vi "intiStage.vi"() -> (0 "error out":errorcluster, 3 "VISA resource name out":refnum<visa-resource-name>)   [LabVIEW 2016]
uses:
  <vilib>/Instr/_visa.llb/VISA Configure Serial Port (Instr).vi
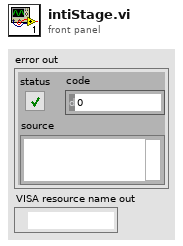
[diagram p1: front panel]
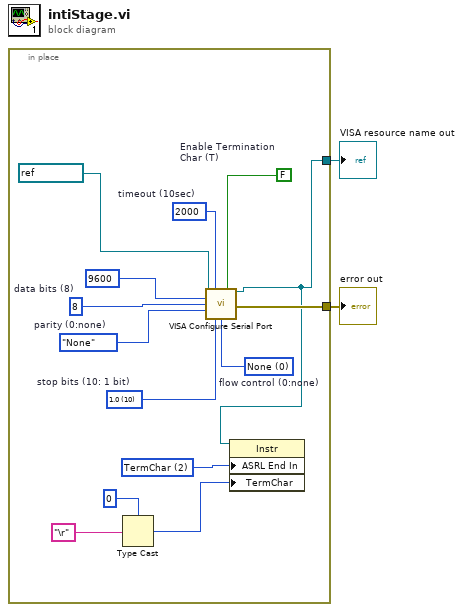
[diagram p0: block diagram]
diagram:
  n1 = in-place {
    in-place-border: [w3] -> w1
    in-place-border: [w8] -> w2
    w4 = u16 2 items=["None", "Last Bit", "TermChar"] ("Serial Settings:End Mode for Reads")
    w10 = u16 0 items=["None", "XON/XOFF", "RTS/CTS", "XON/XOFF & RTS/CTS", "DTR/DSR", "XON/XOFF & DTR/DSR"]  # flow control (0:none)
    w11 = u16 10 items=["1.0"=10, "1.5"=15, "2.0"=20]  # stop bits (10: 1 bit)
    w12 = FALSE  # Enable Termination Char (T)
    w13 = u32 2000  # timeout (10sec)
    w14 = enum16{"None", "Odd", "Even", "Mark", "Space"}."None"  # parity (0:none)
    w15 = u16 8  # data bits (8)
    n2 = Type Cast(type=u8 0, x="\r") -> (*(type *) &x=w6:u8)
    n3 = call-poly "VISA Configure Serial Port"("VISA resource name"=refnum<visa-resource-name> "COM4", "timeout (10sec)"=w13, "Enable Termination\nChar (T)"=w12, "baud rate (9600)"=u32 9600, "data bits (8)"=w15, "parity (0:none)"=w14, "stop bits (10: 1 bit)"=w11, "flow control (0:none)"=w10) -> ("VISA resource name out"=w3:refnum<visa-resource-name>, "error out"=w8:errorcluster)  [unwired: 6 in]
    n4 = property class="Instr"(reference=w3, "ASRL End In"=w4, "TermChar"=w6) -> ()  [unwired: 1 in, 2 out]
  }
  "error out" <- w2
  "VISA resource name out" <- w1
